vi "Pointer.Advanced Copy.vi"() -> ()   [LabVIEW 2016]
uses:
  Source/Classes/Pointer/New (1B).vi
  Source/Classes/Pointer/Write (0D DBL).vi
  Source/Classes/Pointer/Memory.Pointer.Read.0D.U64.vi
  Source/Classes/Pointer/Memory.Pointer.Read.0D.U32.vi
  Source/Classes/Pointer/Memory.Pointer.Read.0D.U16.vi
  Source/Classes/Pointer/Memory.Pointer.Read.0D.U8.vi
  Source/Classes/Pointer/Memory.Pointer.Read.1D.U8.vi
  Source/Classes/Pointer/Pointer.lvclass
panel:
  out "Pointer U64":u64 format="%016x"
  out "Pointer U32":u32 format="%016x"
  out "Pointer U16":u16 format="%016x"
  out "Pointer U8":u8 format="%016x"
  out "Unflatten U64":u64 format="%016x"
  out "Unflatten U32":u32 format="%016x"
  out "Unflatten U16":u16 format="%016x"
  out "Unflatten U8":u8 format="%016x"
  out "Type Cast U64":u64 format="%016x"
  out "Type Cast U32":u32 format="%016x"
  out "Type Cast U16":u16 format="%016x"
  out "Type Cast U8":u8 format="%016x"
  out "Type Cast bytes":string
  in  "stop":bool
  out "Pointer bytes":string
  in  "Advanced Copy dst byte order":enum16{"big-endian", "little-endian"}(ring)
  in  "src width":u64=8 format="%d bytes"
  in  "dst width":u64=4 format="%d bytes"
  out "Flattened string bytes":string
  in  "Flatten to String byte order":T1(ring)
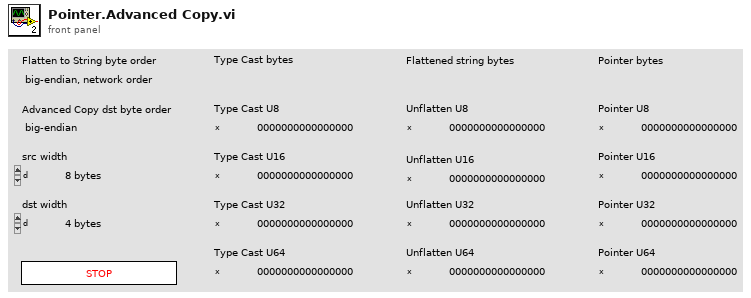
[diagram p1: front panel]
types:
  T1 = enum16{"big-endian, network order", "native, host order", "little-endian"}
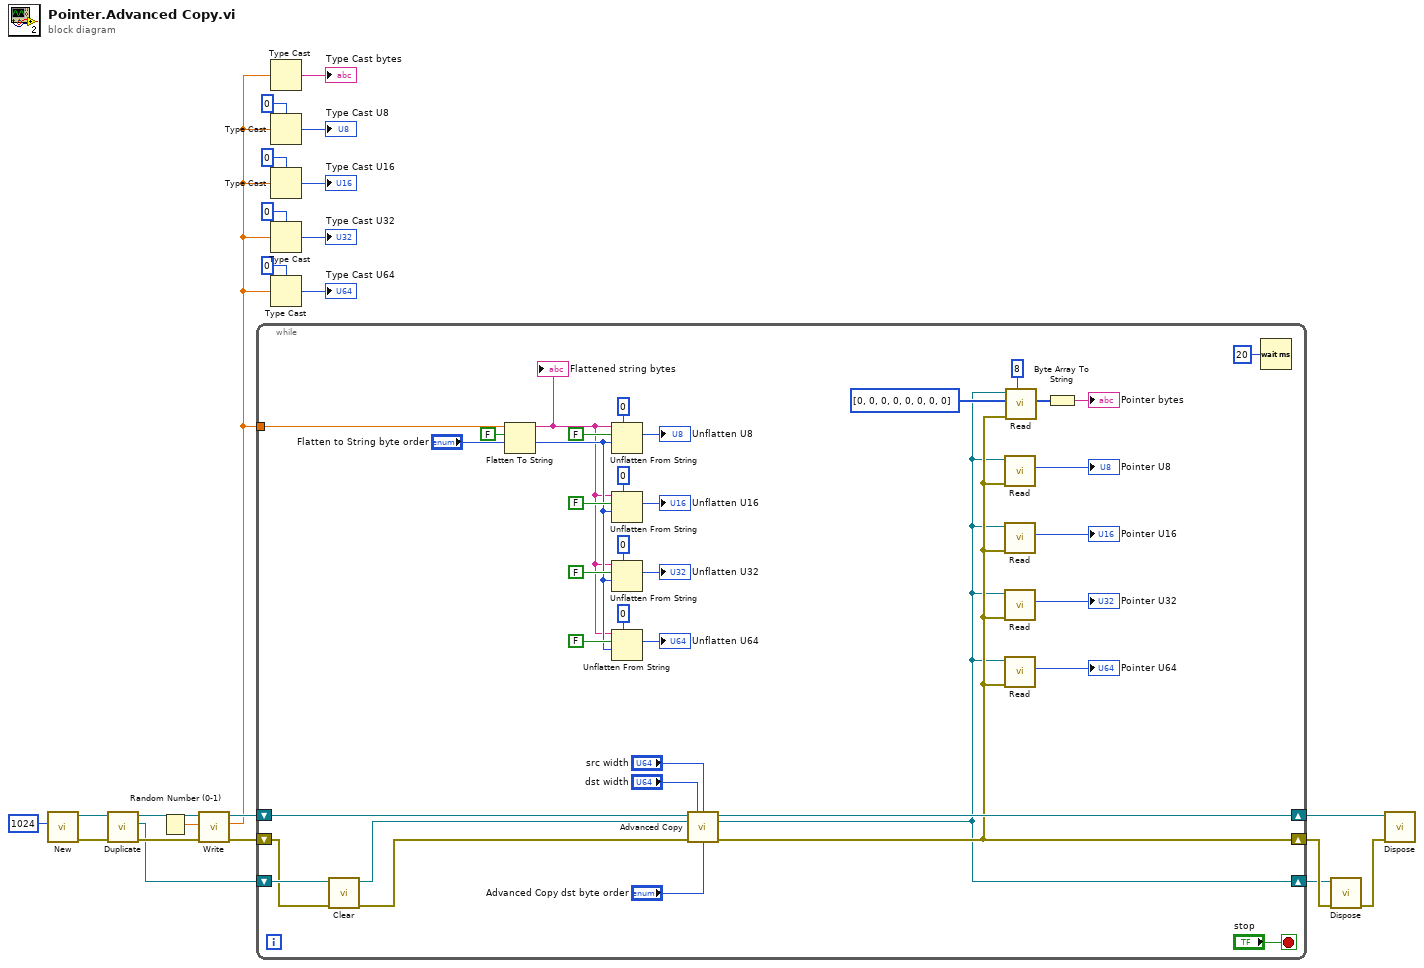
[diagram p0: block diagram]
diagram:
  n1 = call-poly "New.vi"("count (1)"=u64 1024 ("size")) -> ("error out"=w19:errorcluster, "Pointer"=w18:refnum<class "Pointer.lvclass">)  [unwired: 9 in]
  n2 = call "Duplicate.vi"("error in (no error)"=w19, "Pointer in"=w18) -> ("error out"=w16:errorcluster, "new duplicate Pointer"=w15:refnum<class "Pointer.lvclass">, "Pointer out"=w17:refnum<class "Pointer.lvclass">)  [unwired: 7 in]
  n3 = Random Number (0-1)() -> (number: 0 to 1=w22:dbl)
  n4 = call-poly "Write.vi"("error in (no error)"=w16, "value"=w22, "Pointer in"=w17) -> ("error out"=w21:errorcluster, "value"=w8:dbl, "Pointer out"=w20:refnum<class "Pointer.lvclass">)  [unwired: 5 in, 1 out]
  n5 = while {
    tunnel: w8 -> [w51]
    shift-right: [w32] -> w14
    shift-left: w21 -> [w38]
    shift-right: [w57] -> w12
    shift-left: w20 -> [w50]
    shift-right: [w26] -> w11
    shift-left: w15 -> [w52]
    stop <- "stop" stop-if-true
    n6 = call "Clear.vi"("error in (no error)"=w38, "Pointer in"=w52) -> ("error out"=w53:errorcluster, "Pointer out"=w24:refnum<class "Pointer.lvclass">)  [unwired: 8 in]
    n7 = Flatten To String(anything=w51, prepend array or string size? (T)=FALSE, byte order (0:big-endian, network order)="Flatten to String byte order") -> (data string=w39:string)  [unwired: 1 in, 2 out]
    "Flattened string bytes" <- w39
    n8 = Unflatten From String(type=u8 0, binary string=w39, data includes array or string size? (T)=FALSE, byte order (0:big-endian, network order)="Flatten to String byte order") -> (value=→"Unflatten U8":u8)  [unwired: 1 in, 2 out]
    n9 = Unflatten From String(type=u16 0, binary string=w39, data includes array or string size? (T)=FALSE, byte order (0:big-endian, network order)="Flatten to String byte order") -> (value=→"Unflatten U16":u16)  [unwired: 1 in, 2 out]
    n10 = Unflatten From String(type=u32 0, binary string=w39, data includes array or string size? (T)=FALSE, byte order (0:big-endian, network order)="Flatten to String byte order") -> (value=→"Unflatten U32":u32)  [unwired: 1 in, 2 out]
    n11 = Unflatten From String(type=u64 0, binary string=w39, data includes array or string size? (T)=FALSE, byte order (0:big-endian, network order)="Flatten to String byte order") -> (value=→"Unflatten U64":u64)  [unwired: 1 in, 2 out]
    n12 = call "Advanced Copy.vi"("src Pointer in"=w50, "dst width"="dst width", "src width"="src width", "dst Pointer in"=w24, "error in (no error)"=w53, "dst byte order (little-endian)"="Advanced Copy dst byte order") -> ("src Pointer out"=w57:refnum<class "Pointer.lvclass">, "dst Pointer out"=w26:refnum<class "Pointer.lvclass">, "error out"=w32:errorcluster)  [unwired: 7 in]
    n13 = call-poly "Read.vi"("error in (no error)"=w32, "Pointer in"=w26) -> ("value out"=→"Pointer U8":u8)  [unwired: 6 in, 3 out]
    n14 = call-poly "Read.vi"("error in (no error)"=w32, "Pointer in"=w26) -> ("value out"=→"Pointer U16":u16)  [unwired: 6 in, 3 out]
    n15 = call-poly "Read.vi"("error in (no error)"=w32, "Pointer in"=w26) -> ("value out"=→"Pointer U32":u32)  [unwired: 6 in, 3 out]
    n16 = call-poly "Read.vi"("error in (no error)"=w32, "Pointer in"=w26) -> ("value out"=→"Pointer U64":u64)  [unwired: 6 in, 3 out]
    n17 = call-poly "Read.vi"("count (-1: all)"=i64 8, "error in (no error)"=w32, "buffer in"=u8[] [0, 0, 0, 0, 0, 0, 0, 0], "Pointer in"=w26) -> ("buffer out"=w56:u8[])  [unwired: 4 in, 3 out]
    n18 = Byte Array To String(unsigned byte array=w56) -> (string=→"Pointer bytes":string)
    n19 = Wait (ms)(milliseconds to wait=u32 20) -> ()  [unwired: 1 out]
  }
  n20 = Type Cast(x=w8) -> (*(type *) &x=→"Type Cast bytes":string)  [unwired: 1 in]
  n21 = Type Cast(type=u8 0, x=w8) -> (*(type *) &x=→"Type Cast U8":u8)
  n22 = Type Cast(type=u16 0, x=w8) -> (*(type *) &x=→"Type Cast U16":u16)
  n23 = Type Cast(type=u32 0, x=w8) -> (*(type *) &x=→"Type Cast U32":u32)
  n24 = Type Cast(type=u64 0, x=w8) -> (*(type *) &x=→"Type Cast U64":u64)
  n25 = call "Dispose.vi"("error in (no error)"=w14, "Pointer in"=w11) -> ("error out"=w13:errorcluster)  [unwired: 8 in, 1 out]
  n26 = call "Dispose.vi"("error in (no error)"=w13, "Pointer in"=w12) -> ()  [unwired: 8 in, 2 out]
